vi "get_top-level_component_class_name.vi"(8 "error in (no error)":errorcluster, 11 "top-level component type":T1) -> (0 "error out":errorcluster, 2 "component class name":string)   [LabVIEW 2010]
uses:
  common/enumerations/top-level_component_type_enum.ctl
  components/ImagingMode/GenericImagingMode/GenericImagingMode/GenericImagingMode.lvclass
  components/ScanHead/GenericScanHead/GenericScanHead/GenericScanHead.lvclass
  components/DAQ/GenericDAQ/GenericDAQ/GenericDAQ.lvclass
  components/ImageAssembler/GenericImageAssembler/GenericImageAssembler/GenericImageAssembler.lvclass
  components/Display/GenericDisplay/GenericDisplay/GenericDisplay.lvclass
  components/DataCollection/GenericDataCollection/GenericDataCollection/GenericDataCollection.lvclass
  components/Analyser/GenericAnalyser/GenericAnalyser/GenericAnalyser.lvclass
  components/Stimulator/GenericStimulator/GenericStimulator/GenericStimulator.lvclass
  components/ExperimentController/GenericExperimentController/GenericExperimentController/GenericExperimentController.lvclass
  components/Instrument/GenericInstrument/GenericInstrument/GenericInstrument.lvclass
  components/Stage/GenericStage/GenericStage/GenericStage.lvclass
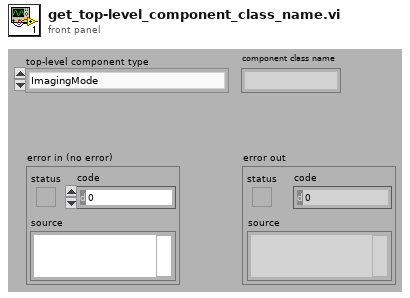
[diagram p1: front panel]
types:
  T1 = typedef "top-level_component_type_enum.ctl" = enum16{"ImagingMode", "ScanHead", "DAQ", "ImageAssembler", "Display", "DataCollection", "Analyser", "Stimulator", "ExperimentController", "Instrument", "Stage"}
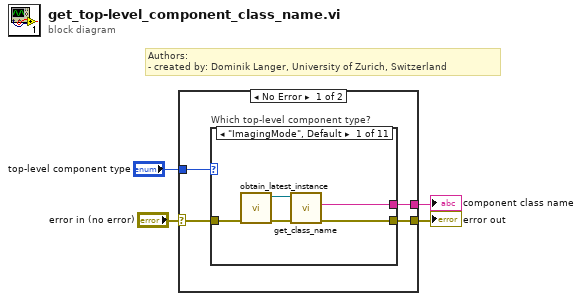
[diagram p0: block diagram]
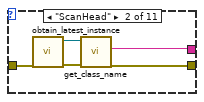
[diagram p2: hidden frame]
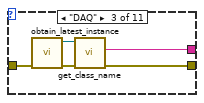
[diagram p3: hidden frame]
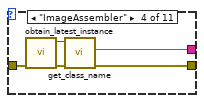
[diagram p4: hidden frame]
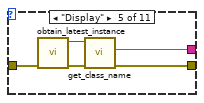
[diagram p5: hidden frame]
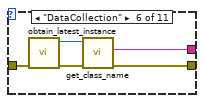
[diagram p6: hidden frame]
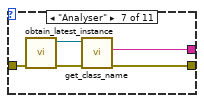
[diagram p7: hidden frame]
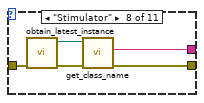
[diagram p8: hidden frame]
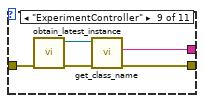
[diagram p9: hidden frame]
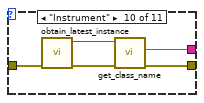
[diagram p10: hidden frame]
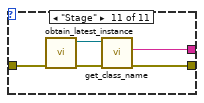
[diagram p11: hidden frame]
diagram:
  # "Authors: \n- created by: Dominik Langer, University of Zurich, Switzerland"
  n1 = case shown="No Error" "error in (no error)" {
    selector: "error in (no error)" -> [w7 w64]
    tunnel: "top-level component type" -> [w8 _]
    tunnel: [w6 w64] -> w2
    tunnel: [w5 _] -> w1
    frame No Error {
      n2 = case "Which top-level component type?" shown="\"ImagingMode\", Default" w8 {
        tunnel: w7 -> [w13 w18 w23 w28 w33 w38 w43 w48 w53 w58 w63]
        tunnel: [w10 w15 w20 w25 w30 w35 w41 w46 w51 w55 w60] -> w6
        tunnel: [w12 w14 w19 w24 w29 w34 w40 w44 w50 w54 w59] -> w5
        frame "ImagingMode", Default {
          n3 = call "obtain_latest_instance.vi"("error in (no error)"=w13) -> ("error out"=w11:errorcluster, "GenericScanMode out"=w9:refnum<class "GenericImagingMode.lvclass">)  [unwired: 9 in]
          n4 = call-dynamic "get_class_name.vi"("error in (no error)"=w11, "GenericPlugin in"=w9) -> ("error out"=w10:errorcluster, "class name"=w12:string)  [unwired: 5 in, 3 out]
        }
        frame "ScanHead" {
          n5 = call "obtain_latest_instance.vi"("error in (no error)"=w18) -> ("error out"=w17:errorcluster, "GenericScanHead out"=w16:refnum<class "GenericScanHead.lvclass">)  [unwired: 9 in]
          n6 = call-dynamic "get_class_name.vi"("error in (no error)"=w17, "GenericPlugin in"=w16) -> ("error out"=w15:errorcluster, "class name"=w14:string)  [unwired: 5 in, 3 out]
        }
        frame "DAQ" {
          n7 = call "obtain_latest_instance.vi"("error in (no error)"=w23) -> ("error out"=w22:errorcluster, "GenericDAQ out"=w21:refnum<class "GenericDAQ.lvclass">)  [unwired: 9 in]
          n8 = call-dynamic "get_class_name.vi"("error in (no error)"=w22, "GenericPlugin in"=w21) -> ("error out"=w20:errorcluster, "class name"=w19:string)  [unwired: 5 in, 3 out]
        }
        frame "ImageAssembler" {
          n9 = call "obtain_latest_instance.vi"("error in (no error)"=w28) -> ("error out"=w27:errorcluster, "GenericImageAssembler out"=w26:refnum<class "GenericImageAssembler.lvclass">)  [unwired: 9 in]
          n10 = call-dynamic "get_class_name.vi"("error in (no error)"=w27, "GenericPlugin in"=w26) -> ("error out"=w25:errorcluster, "class name"=w24:string)  [unwired: 5 in, 3 out]
        }
        frame "Display" {
          n11 = call "obtain_latest_instance.vi"("error in (no error)"=w33) -> ("error out"=w32:errorcluster, "GenericDisplay out"=w31:refnum<class "GenericDisplay.lvclass">)  [unwired: 9 in]
          n12 = call-dynamic "get_class_name.vi"("error in (no error)"=w32, "GenericPlugin in"=w31) -> ("error out"=w30:errorcluster, "class name"=w29:string)  [unwired: 5 in, 3 out]
        }
        frame "DataCollection" {
          n13 = call "obtain_latest_instance.vi"("error in (no error)"=w38) -> ("error out"=w37:errorcluster, "GenericDataCollection out"=w36:refnum<class "GenericDataCollection.lvclass">)  [unwired: 9 in]
          n14 = call-dynamic "get_class_name.vi"("error in (no error)"=w37, "GenericPlugin in"=w36) -> ("error out"=w35:errorcluster, "class name"=w34:string)  [unwired: 5 in, 3 out]
        }
        frame "Analyser" {
          n15 = call "obtain_latest_instance.vi"("error in (no error)"=w43) -> ("error out"=w42:errorcluster, "GeneralAnalyser out"=w39:refnum<class "GenericAnalyser.lvclass">)  [unwired: 9 in]
          n16 = call-dynamic "get_class_name.vi"("error in (no error)"=w42, "GenericPlugin in"=w39) -> ("error out"=w41:errorcluster, "class name"=w40:string)  [unwired: 5 in, 3 out]
        }
        frame "Stimulator" {
          n17 = call "obtain_latest_instance.vi"("error in (no error)"=w48) -> ("error out"=w47:errorcluster, "GenericStimulator out"=w45:refnum<class "GenericStimulator.lvclass">)  [unwired: 9 in]
          n18 = call-dynamic "get_class_name.vi"("error in (no error)"=w47, "GenericPlugin in"=w45) -> ("error out"=w46:errorcluster, "class name"=w44:string)  [unwired: 5 in, 3 out]
        }
        frame "ExperimentController" {
          n19 = call "obtain_latest_instance.vi"("error in (no error)"=w53) -> ("error out"=w52:errorcluster, "GenericExperimentController out"=w49:refnum<class "GenericExperimentController.lvclass">)  [unwired: 9 in]
          n20 = call-dynamic "get_class_name.vi"("error in (no error)"=w52, "GenericPlugin in"=w49) -> ("error out"=w51:errorcluster, "class name"=w50:string)  [unwired: 5 in, 3 out]
        }
        frame "Instrument" {
          n21 = call "obtain_latest_instance.vi"("error in (no error)"=w58) -> ("error out"=w57:errorcluster, "microscope"=w56:refnum<class "GenericInstrument.lvclass">)  [unwired: 9 in]
          n22 = call-dynamic "get_class_name.vi"("error in (no error)"=w57, "GenericPlugin in"=w56) -> ("error out"=w55:errorcluster, "class name"=w54:string)  [unwired: 5 in, 3 out]
        }
        frame "Stage" {
          n23 = call "obtain_latest_instance.vi"("error in (no error)"=w63) -> ("error out"=w62:errorcluster, "GenericStage out"=w61:refnum<class "GenericStage.lvclass">)  [unwired: 9 in]
          n24 = call-dynamic "get_class_name.vi"("error in (no error)"=w62, "GenericPlugin in"=w61) -> ("error out"=w60:errorcluster, "class name"=w59:string)  [unwired: 5 in, 3 out]
        }
      }
    }
    frame Error {
    }
  }
  "error out" <- w2
  "component class name" <- w1
